vi "create.vi"(8 "error in (no error)":errorcluster, 11 "StringGeneratorAK110125StimServerCmd in":refnum<class "StringGeneratorAK110125StimServerCmd.lvclass">) -> (0 "error out":errorcluster, 2 "string":string, 3 "StringGeneratorAK110125StimServerCmd out":refnum<class "StringGeneratorAK110125StimServerCmd.lvclass">)   [LabVIEW 2010, in "StringGeneratorAK110125StimServerCmd.lvclass"]
uses:
  StringGeneratorAK110125StimServerCmd.lvclass
  StringGeneratorAK110125StimServerCmd.lvclass/StringGeneratorAK110125StimServerCmd.ctl
  <vilib>/gmath/statdist.llb/Random Permutation.vi
  <vilib>/gmath/NI_Gmath.lvlib
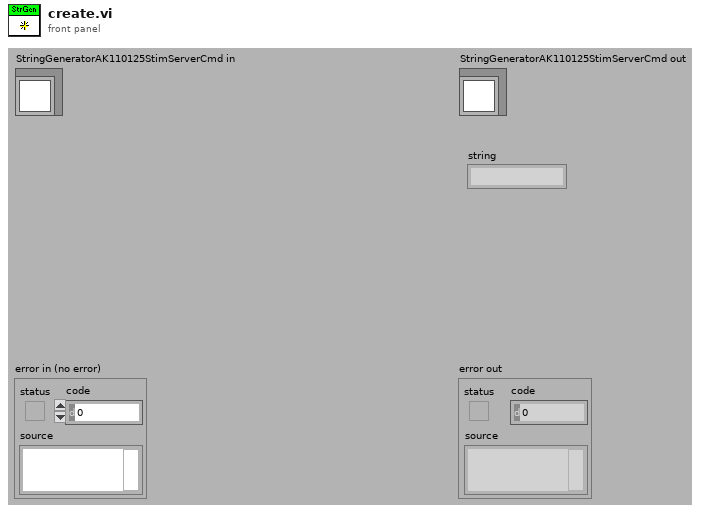
[diagram p1: front panel]
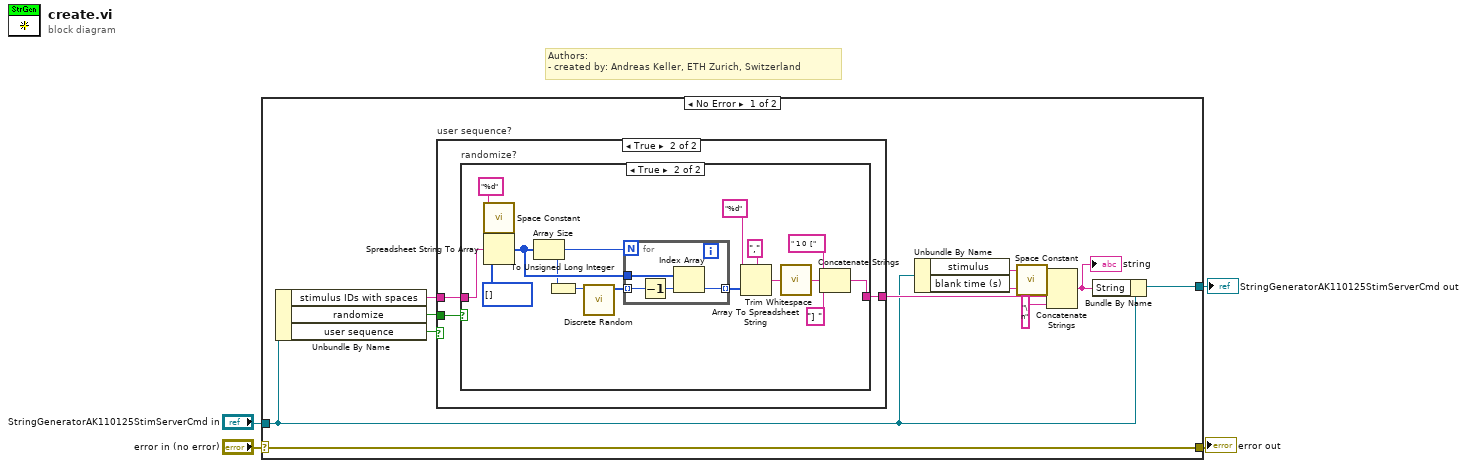
[diagram p0: block diagram]
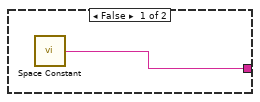
[diagram p2: hidden frame]
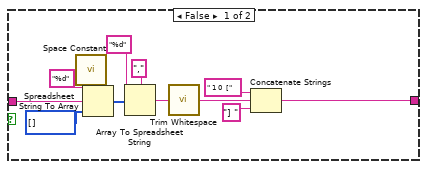
[diagram p3: hidden frame]
diagram:
  # "Authors: \n- created by: Andreas Keller, ETH Zurich, Switzerland"
  n1 = case shown="No Error" "error in (no error)" {
    selector: "error in (no error)" -> [w13 w54]
    tunnel: [w13 w54] -> w4
    tunnel: [w12 w53] -> w3
    tunnel: "StringGeneratorAK110125StimServerCmd in" -> [w10 w53]
    frame No Error {
      n2 = Unbundle By Name(w10) -> ("stimulus IDs with spaces"=w11:string, "randomize"=w7:bool, "user sequence"=w6:bool)
      n3 = case "user sequence?" shown="True" w6 {
        tunnel: [w17 w19] -> w16
        tunnel: w7 -> [_ w20]
        tunnel: w11 -> [_ w18]
        frame False {
          n4 = call <vilib>:"Space Constant.vi"() -> ("String"=w17:string)
        }
        frame True {
          n5 = case "randomize?" shown="True" w20 {
            tunnel: [w21 w34] -> w19
            tunnel: w18 -> [w22 w33]
            frame False {
              n6 = call <vilib>:"Space Constant.vi"() -> ("String"=w31:string)
              n7 = Spreadsheet String To Array(delimiter (Tab)=w31, format string="%d", spreadsheet string=w22, array type (2D Dbl)=u32[] []) -> (array=w32:u32[])
              n8 = Array To Spreadsheet String(delimiter (Tab)=",", array=w32, 3:"%d" ("format string")) -> (spreadsheet string=w26:string)
              n9 = call <vilib>:"Trim Whitespace.vi"("string"=w26) -> ("trimmed string"=w25:string)  [unwired: 1 in]
              n10 = Concatenate Strings(" 1 0  [" ("string"), w25, "] " ("string")) -> (w21:string)
            }
            frame True {
              n11 = call <vilib>:"Space Constant.vi"() -> ("String"=w35:string)
              n12 = Spreadsheet String To Array(delimiter (Tab)=w35, format string="%d", spreadsheet string=w33, array type (2D Dbl)=u32[] []) -> (array=w41:u32[])
              n13 = Array Size(array=w41) -> (size(s)=w39:i32)
              n14 = To Unsigned Long Integer(number=w39) -> (unsigned 32bit integer=w38:u32)
              n15 = call-poly <vilib>:"Discrete Random.vi"("N"=w38) -> ("random permutation"=w40:i32[])  [unwired: 9 in, 1 out]
              n16 = for {
                N: w39 -> [_]
                tunnel: w40 -> [w52] mode=indexing
                tunnel: w41 -> [w50]
                tunnel: [w49] -> w42 mode=indexing
                n17 = Decrement(x=w52) -> (x-1=w51:i32)
                n18 = Index Array(array=w50, index=w51) -> (element=w49:u32)
              }
              n19 = Array To Spreadsheet String(delimiter (Tab)=",", array=w42, 3:"%d" ("format string")) -> (spreadsheet string=w45:string)
              n20 = call <vilib>:"Trim Whitespace.vi"("string"=w45) -> ("trimmed string"=w46:string)  [unwired: 1 in]
              n21 = Concatenate Strings(" 1 0  [" ("string"), w46, "] " ("string")) -> (w34:string)
            }
          }
        }
      }
      n22 = Unbundle By Name(w10) -> ("stimulus"=w9:string, "blank time (s)"=w8:string)
      n23 = call <vilib>:"Space Constant.vi"() -> ("String"=w15:string)
      n24 = Concatenate Strings(w9, w15, w8, w16, "\n" ("string")) -> (w5:string)
      "string" <- w5
      n25 = Bundle By Name(cluster=w10, "String"=w5) -> (w12:refnum<class "StringGeneratorAK110125StimServerCmd.lvclass">)
    }
    frame Error {
    }
  }
  "error out" <- w4
  "StringGeneratorAK110125StimServerCmd out" <- w3
